vi "DQMH System Message - Get Module Identifier.vi"(8 "error in (no error)":errorcluster, 10 "Module Path":path, 11 "VI Ref":refnum<vi>) -> (0 "error out":errorcluster, 3 "Module Identifier":string)   [LabVIEW 2022 SP3, in "hse-dqmh.lvlib"]
doc: "____\nHAMPEL SOFTWARE ENGINEERING v3.8.0 (2023-12-18 14:41)"
uses:
  hse-dqmh.lvlib
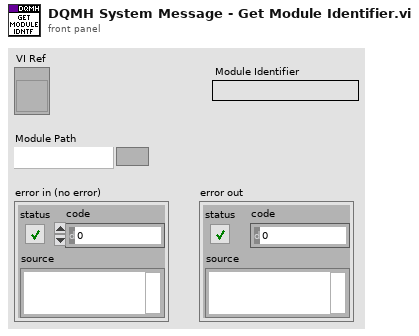
[diagram p1: front panel]
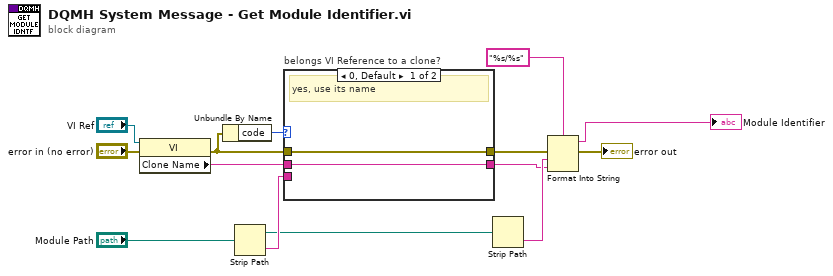
[diagram p0: block diagram]
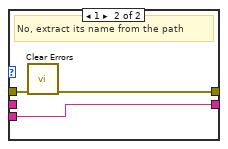
[diagram p2: hidden frame]
diagram:
  n1 = property class="VI"(reference="VI Ref", error in="error in (no error)") -> (error out=w8:errorcluster, "Clone Name"=w13:string)  [unwired: 1 out]
  n2 = Unbundle By Name(w8) -> ("code"=w7:i32)
  n3 = Strip Path(path="Module Path") -> (stripped path=w12:path, name=w14:string)
  n4 = case "belongs VI Reference to a clone?" shown="0, Default" w7 {
    tunnel: [w16 w19] -> w4
    tunnel: w13 -> [w16 _]
    tunnel: w14 -> [_ w19]
    tunnel: [w15 w17] -> w3
    tunnel: w8 -> [w15 w18]
    frame 0, Default {
      # "yes, use its name"
    }
    frame 1 {
      # "No, extract its name from the path"
      n5 = call <vilib>:"Clear Errors.vi"("error in (no error)"=w18) -> ("error out"=w17:errorcluster)  [unwired: 5 in, 1 out]
    }
  }
  n6 = Strip Path(path=w12) -> (name=w5:string)  [unwired: 1 out]
  n7 = Format Into String(format string="%s/%s", error in=w3, w5, w4) -> (resulting string=→"Module Identifier":string, error out=→"error out":errorcluster)  [unwired: 1 in]
